vi "Group_FromEasyObj.vi"(8 "error in (no error)":errorcluster, 11 "input cluster":T1 {"Channels"."Data Reference" format="%.0x"}) -> (0 "error out":errorcluster, 3 "Group out":refnum<class "Group.lvclass">)   [LabVIEW 2023, in "Group.lvclass"]
doc: "Create the group definition given a cluster data representation of it."
uses:
  Group.lvclass
  GroupAsCluster.ctl
  Channel/ChannelAsCluster.ctl
  <vilib>/NI VeriStand/Custom Device API/Data Reference.ctl
  Meta Data.ctl
  Group.lvclass/Group.ctl
  Channel/Channel.lvclass
  <vilib>/NI VeriStand/Custom Device API/Custom Device API.lvlib
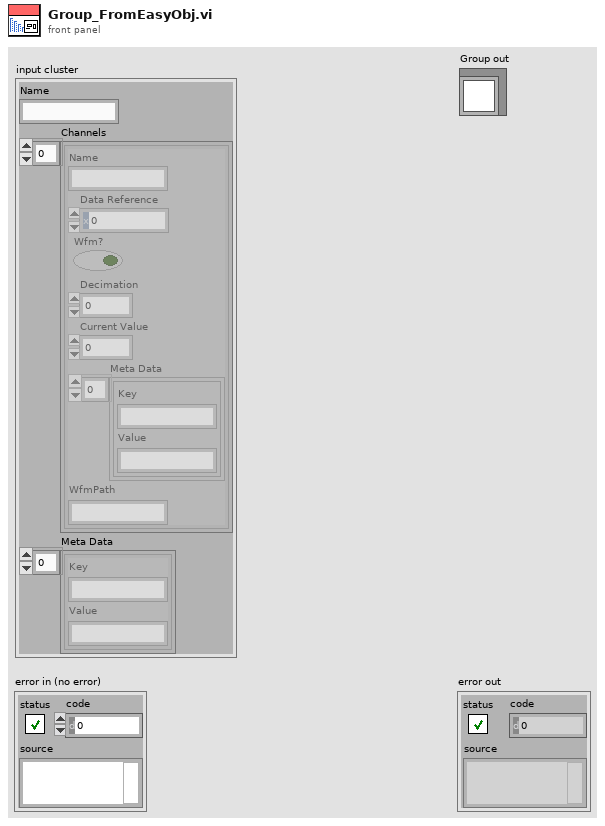
[diagram p1: front panel]
types:
  T1 = typedef "GroupAsCluster.ctl" = cluster{"Name":string, "Channels":T2[], "Meta Data":T4[]}
  T2 = typedef "ChannelAsCluster.ctl" = cluster{"Name":string, "Data Reference":T3, "Wfm?":bool, "Decimation":i32, "Current Value":dbl, "Meta Data":T4[], "WfmPath":string}
  T3 = typedef "Custom Device API.lvlib/Data Reference.ctl" = i32
  T4 = typedef "Meta Data.ctl" = cluster{"Key":string, "Value":string}
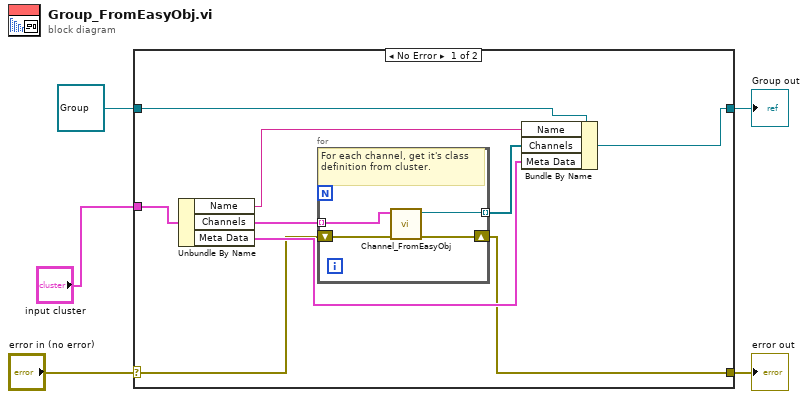
[diagram p0: block diagram]
diagram:
  n1 = case shown="No Error" "error in (no error)" {
    selector: "error in (no error)" -> [w6 w20]
    tunnel: [w8 w20] -> w4
    tunnel: [w13 w19] -> w2
    tunnel: refnum<class "Group.lvclass"> refnum ("Group in") -> [w14 w19]
    tunnel: "input cluster" -> [w12 _]
    frame No Error {
      n2 = Unbundle By Name(w12) -> ("Name"=w11:string, "Channels"=w9:T2[], "Meta Data"=w10:T4[])
      n3 = for {
        tunnel: w9 -> [w18] mode=indexing
        shift-right: [w16] -> w8
        shift-left: w6 -> [w17]
        tunnel: [w15] -> w7 mode=indexing
        # "For each channel, get it's class definition from cluster."
        n4 = call "Channel_FromEasyObj.vi"("error in (no error)"=w17, "output cluster"=w18) -> ("error out"=w16:errorcluster, "Channel out"=w15:refnum<class "Channel.lvclass">)  [unwired: 8 in]
      }
      n5 = Bundle By Name(cluster=w14, "Name"=w11, "Channels"=w7, "Meta Data"=w10) -> (w13:refnum<class "Group.lvclass">)
    }
    frame Error {
    }
  }
  "error out" <- w4
  "Group out" <- w2
